vi "GetConfiguration.vi"(8 "error in (no error)":errorcluster, 11 "Module ID":i32=-1) -> (0 "error out":errorcluster, 1 "timed out?":bool, 2 "Reply Payload":T1)   [LabVIEW 2014, in "Configurable.lvlib"]
doc: "_____\nCreated using Delacor QMH Event Scripter 4.0.0.68."
uses:
  Configurable.lvlib
  GetConfiguration (Reply Payload)--cluster.ctl
  ModuleConfiguration--Cluster.ctl
  GetConfiguration Argument--cluster.ctl
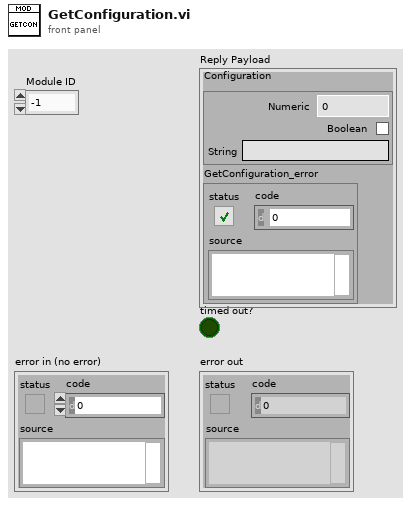
[diagram p1: front panel]
types:
  T1 = typedef "Configurable.lvlib/GetConfiguration (Reply Payload)--cluster.ctl" = cluster{"Configuration":T2, "GetConfiguration_error":errorcluster}
  T2 = typedef "Configurable.lvlib/ModuleConfiguration--Cluster.ctl" = cluster{"Numeric":dbl, "Boolean":bool, "String":string}
  T3 = typedef "Configurable.lvlib/GetConfiguration Argument--cluster.ctl" = cluster{"Module ID":i32, "Wait Notifier":refnum<notifier>}
  T4 = typedef "Configurable.lvlib/Request Events--cluster.ctl" = cluster{"Stop Module":refnum<user-event>, "Show Panel":refnum<user-event>, "Hide Panel":refnum<user-event>, "Show Diagram":refnum<user-event>, "Get Module Execution Status":refnum<user-event>, "GetQualifiedName":refnum<user-event>, "GetConfiguration":refnum<user-event>}
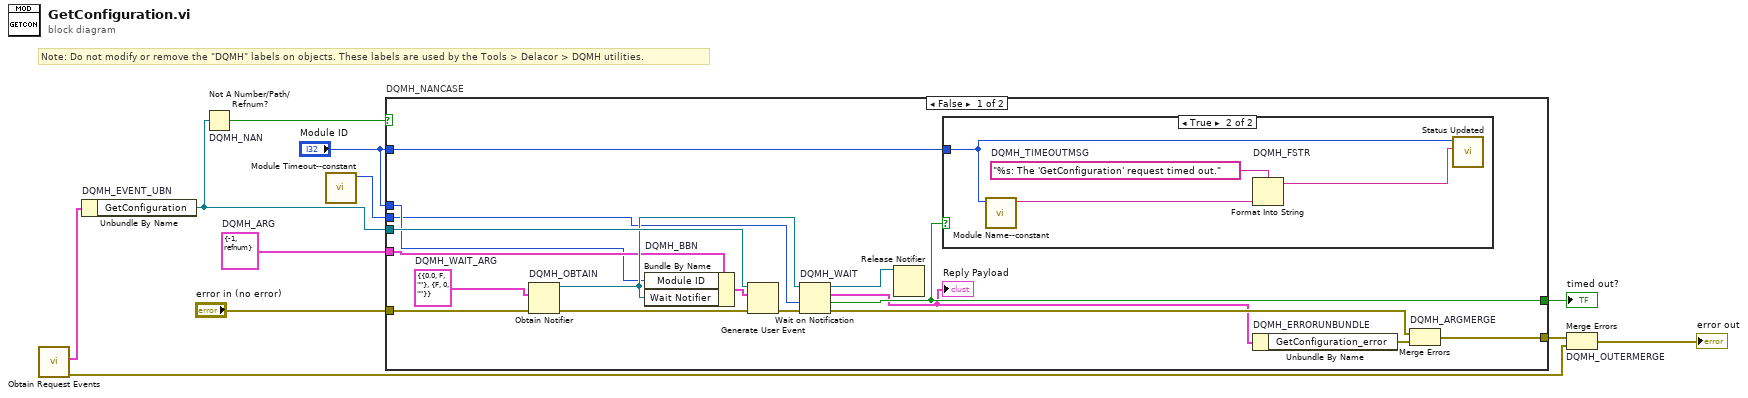
[diagram p0: block diagram]
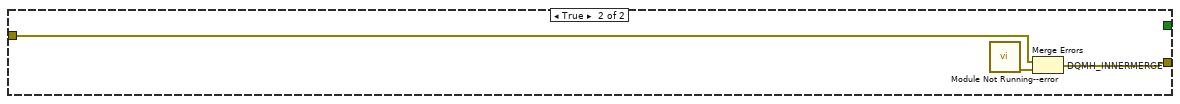
[diagram p3: hidden frame]
diagram:
  w5 = T3 {"Module ID"=-1, "Wait Notifier"=refnum}  # DQMH_ARG
  # "Note: Do not modify or remove the \"DQMH\" labels on objects. These labels are used by the Tools > Delacor > DQMH utilities."
  n1 = call "Obtain Request Events.vi"() -> ("error out"=w2:errorcluster, "Configurable Request Events"=w1:T4)  [unwired: 10 in]
  n2 = Unbundle By Name "DQMH_EVENT_UBN"(w1) -> ("GetConfiguration"=w9:refnum<user-event>)
  n3 = Not A Number/Path/Refnum? "DQMH_NAN"(number/path/refnum=w9) -> (NaN/Path/Refnum?=w8:bool)
  n4 = call "Module Timeout--constant.vi"() -> ("Module Timeout"=w4:i32)  [unwired: 11 in]
  n5 = case "DQMH_NANCASE" shown="False" w8 {
    tunnel: "error in (no error)" -> [w28 w35]
    tunnel: w9 -> [w26 _]
    tunnel: [w19 w34] -> w6
    tunnel: [w20 _] -> w7
    tunnel: w5 -> [w15 _]
    tunnel: "Module ID" -> [w14 _]
    tunnel: w4 -> [w13 _]
    tunnel: "Module ID" -> [w12 _]
    frame False {
      w24 = T1 {"Configuration"={"Numeric"=0.0, "Boolean"=FALSE, "String"=""}, "GetConfiguration_error"={"status"=FALSE, "code"=0, "source"=""}}  # DQMH_WAIT_ARG
      n6 = Obtain Notifier "DQMH_OBTAIN"(notification data type=w24, error in (no error)=w28) -> (notifier out=w22:refnum<notifier>, error out=w25:errorcluster)  [unwired: 2 in, 1 out]
      n7 = Bundle By Name "DQMH_BBN"(cluster=w15, "Module ID"=w14, "Wait Notifier"=w22) -> (w16:T3)
      n8 = Generate User Event(user event=w26, event data cluster=w16, error in=w25) -> (error out=w27:errorcluster)  [unwired: 1 in, 1 out]
      n9 = Wait on Notification "DQMH_WAIT"(notifier=w22, timeout in ms (-1)=w13, error in (no error)=w27) -> (notifier out=w21:refnum<notifier>, notification=w17:T1, timed out?=w20:bool, error out=w23:errorcluster)  [unwired: 1 in]
      "Reply Payload" <- w17
      n10 = Release Notifier(notifier=w21) -> ()  [unwired: 2 in, 3 out]
      n11 = case shown="True" w20 {
        tunnel: w12 -> [_ w29]
        frame False {
        }
        frame True {
          w32 = "%s: The 'GetConfiguration' request timed out."  # DQMH_TIMEOUTMSG
          n12 = call "Module Name--constant.vi"("Module ID"=w29) -> ("Module Name"=w31:string)  [unwired: 10 in]
          n13 = Format Into String "DQMH_FSTR"(format string=w32, w31) -> (resulting string=w30:string)  [unwired: 2 in, 1 out]
          n14 = call "Status Updated.vi"("Status"=w30, "Module ID"=w29) -> ()  [unwired: 9 in, 1 out]
        }
      }
      n15 = Unbundle By Name "DQMH_ERRORUNBUNDLE"(w17) -> ("GetConfiguration_error"=w18:errorcluster)
      n16 = Merge Errors "DQMH_ARGMERGE"(w23, w18) -> (w19:errorcluster)
    }
    frame True {
      n17 = call "Module Not Running--error.vi"() -> ("error out"=w33:errorcluster)  [unwired: 11 in]
      n18 = Merge Errors "DQMH_INNERMERGE"(w35, w33) -> (w34:errorcluster)
    }
  }
  "timed out?" <- w7
  n19 = Merge Errors "DQMH_OUTERMERGE"(w6, w2) -> (→"error out":errorcluster)
